vi "Logger.Stats.UpdateGraph.vi"(8 "error in (no error)":errorcluster, 9 "Selection":i32[](array[numeric]), 10 "Results":T1[](array[typedef]) {"Time From" format="%<%X %x>T"; "Time To" format="%<%X %x>T"}, 11 "Graph":refnum<vi>) -> (0 "error out":errorcluster)   [LabVIEW 2016]
uses:
  Logger.Stats.Fglb.Result.ctl
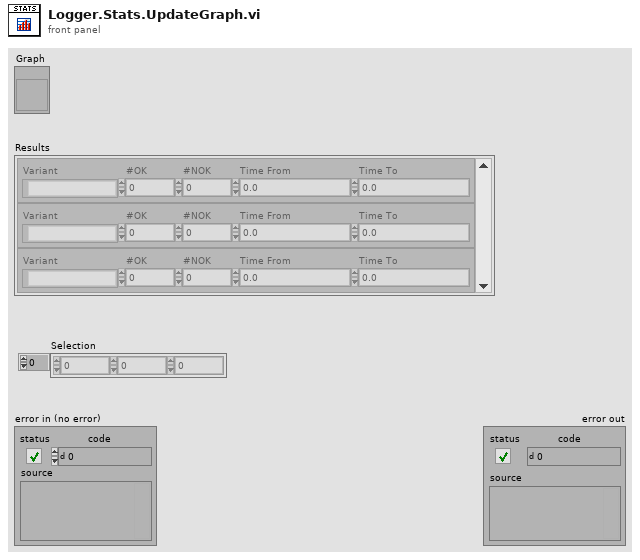
[diagram p1: front panel]
types:
  T1 = typedef "Logger.Stats.Fglb.Result.ctl" = cluster{"Variant":string, "#OK":i32, "#NOK":i32, "Time From":dbl, "Time To":dbl}
  T2 = cluster{"Name":string, "Color":u32, "Style":i32, "Point Style":i32, "Name Visible":bool, "Allow Drag":bool, "Annotation Mode":u32, "Plot":i32, "Index":i32, "Position":cluster{"X":dbl, "Y":dbl}, "X Scale":i32, "Y Scale":u32, "Show Arrow":bool, "Lock Name":bool, "Plot Area":i32, "Label Offset":cluster{"X":dbl, "Y":i32}}
  T3 = cluster{"Name":string, "Color":u32, "Style":i32, "Point Style":i32, "Name Visible":bool, "Allow Drag":bool, "Annotation Mode":u32, "Plot":i32, "Index":i32, "Position":cluster{"X":dbl, "Y":dbl}, "X Scale":i32, "Y Scale":u32, "Show Arrow":bool, "Lock Name":bool, "Plot Area":i32, "Label Offset":cluster{"X":dbl, "Y":i32}}[]
  T4 = typedef "LVAnnotationListTypeDef.ctl" = cluster{"Name":string, "Color":u32, "Style":u8, "Point Style":u8, "Name Visible":bool, "Allow Drag":bool, "Annotation Mode":u32, "Plot":i32, "Index":i32, "Position":cluster{"X":dbl, "Y":dbl}, "X Scale":u32, "Y Scale":u32, "Show Arrow":bool, "Lock Name":bool, "Plot Area":i32, "Label Offset":cluster{"X":dbl, "Y":dbl}}[]
  T5 = cluster{"Name":string, "Color":u32, "Style":u8, "Point Style":u8, "Name Visible":bool, "Allow Drag":bool, "Annotation Mode":u32, "Plot":i32, "Index":i32, "Position":cluster{"X":dbl, "Y":dbl}, "X Scale":u32, "Y Scale":u32, "Show Arrow":bool, "Lock Name":bool, "Plot Area":i32, "Label Offset":cluster{"X":dbl, "Y":dbl}}
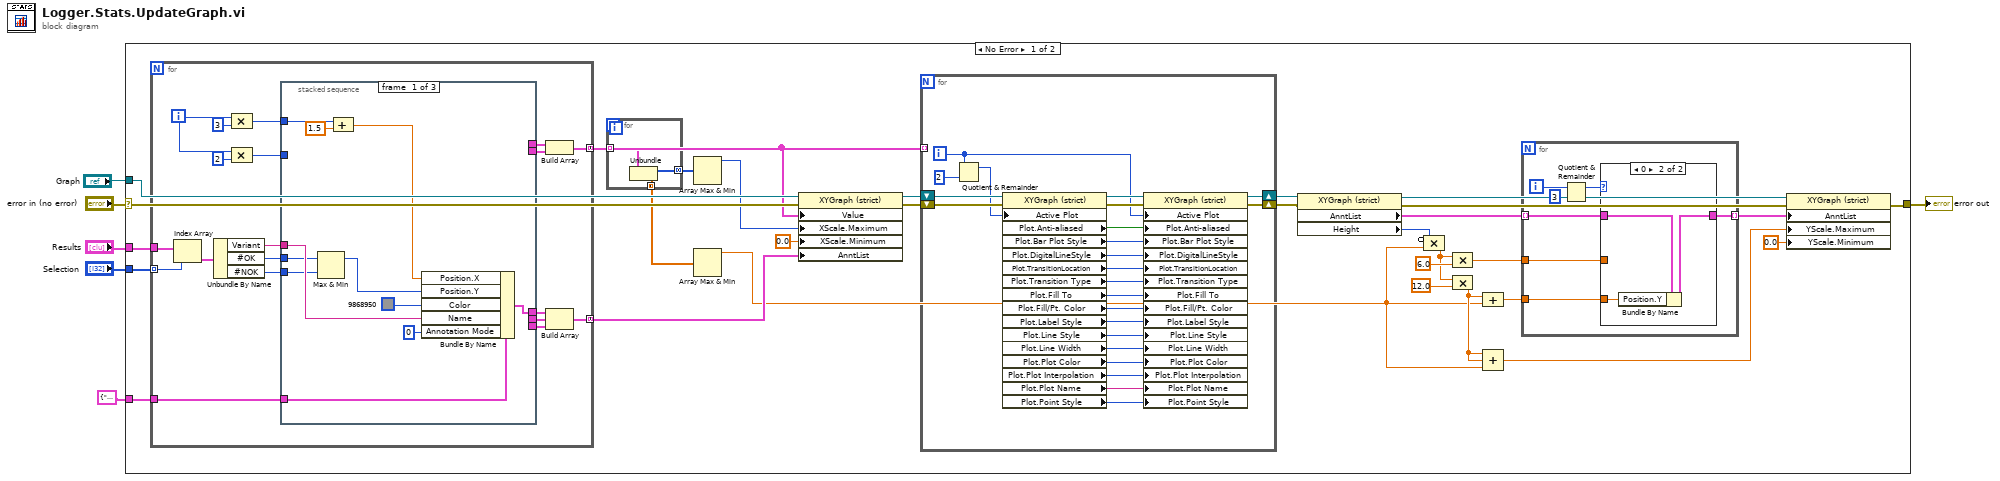
[diagram p0: block diagram]
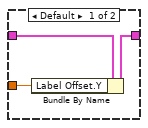
[diagram p2: hidden frame]
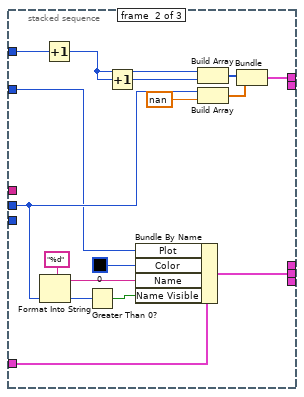
[diagram p3: hidden frame]
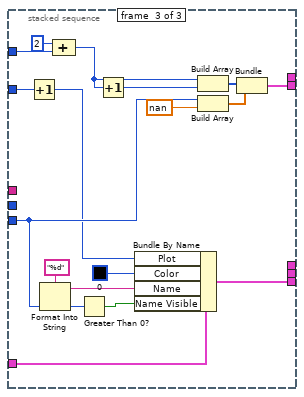
[diagram p4: hidden frame]
diagram:
  n1 = case shown="No Error" "error in (no error)" {
    selector: "error in (no error)" -> [w34 w138]
    tunnel: [w24 w138] -> w5
    tunnel: "Results" -> [w36 _]
    tunnel: "Graph" -> [w33 _]
    tunnel: "Selection" -> [w35 _]
    tunnel: T2 {"Name"="", "Color"=0, "Style"=0, "Point Style"=0, "Name Visible"=TRUE, "Allow Drag"=FALSE, "Annotation Mode"=1, "Plot"=0, "Index"=0, "Position"={"X"=0.0, "Y"=0.0}, "X Scale"=0, "Y Scale"=0, "Show Arrow"=FALSE, "Lock Name"=TRUE, "Plot Area"=0, "Label Offset"={"X"=0.0, "Y"=0}} ("Cluster") -> [w32 _]
    frame No Error {
      n2 = for {
        tunnel: w36 -> [w68]
        tunnel: w35 -> [w67] mode=indexing
        tunnel: w32 -> [w63]
        tunnel: [w55] -> w30 mode=concatenating
        tunnel: [w56] -> w25 mode=concatenating
        i -> [w52]
        n3 = Index Array(array=w68, index=w67) -> (element=w66:T1)
        n4 = Unbundle By Name(w66) -> ("Variant"=w57:string, "#OK"=w64:i32, "#NOK"=w54:i32)
        n5 = Compound Arithmetic op=MULTIPLY(w52, 3 ("value")) -> (w62:i32)
        n6 = Compound Arithmetic op=MULTIPLY(w52, 2 ("value")) -> (w51:i32)
        n7 = stacked-sequence {
          tunnel: w64 -> [w71 w83 _]
          tunnel: w54 -> [w70 _ w101]
          tunnel: w63 -> [w78 w93 w110]
          tunnel: w62 -> [w74 w90 w97]
          tunnel: [_ w85 _] -> w60
          tunnel: [_ w84 _] -> w61
          tunnel: [_ _ w104] -> w59
          tunnel: [_ _ w103] -> w58
          tunnel: w57 -> [w77 _ _]
          tunnel: w51 -> [_ w80 w99]
          tunnel: [w76 _ _] -> w50
          frame #0 {
            n8 = Max & Min(x=w71, y=w70) -> (max(x,y)=w69:i32)  [unwired: 1 out]
            n9 = Compound Arithmetic op=unknown(w74, 1.5 ("value")) -> (w72:dbl)
            n10 = Bundle By Name(cluster=w78, "Position.X"=w72, "Position.Y"=w69, "Color"=u32 9868950, "Name"=w77, "Annotation Mode"=u32 0) -> (w76:T2)
          }
          frame #1 {
            n11 = Format Into String(format string="%d", w83) -> (resulting string=w91:string)  [unwired: 2 in, 1 out]
            n12 = Increment(x=w90) -> (x+1=w81:i32)
            n13 = Greater Than 0?(x=w83) -> (x > 0?=w82:bool)
            n14 = Increment(x=w81) -> (x+1=w89:i32)
            n15 = Bundle By Name(cluster=w93, "Plot"=w80, "Color"=u32 0, "Name"=w91, "Name Visible"=w82) -> (w84:T2)
            n16 = Build Array(w81, w89) -> (w87:i32[])
            n17 = Build Array(w83, nan ("element")) -> (w86:dbl[])
            n18 = Bundle(w87, w86) -> (w85:cluster{i32[], dbl[]})  [unwired: 1 in]
          }
          frame #2 {
            n19 = Increment(x=w99) -> (x+1=w98:i32)
            n20 = Format Into String(format string="%d", w101) -> (resulting string=w108:string)  [unwired: 2 in, 1 out]
            n21 = Compound Arithmetic op=ADD(2 ("value"), w97) -> (w95:i32)
            n22 = Greater Than 0?(x=w101) -> (x > 0?=w102:bool)
            n23 = Increment(x=w95) -> (x+1=w100:i32)
            n24 = Bundle By Name(cluster=w110, "Plot"=w98, "Color"=u32 0, "Name"=w108, "Name Visible"=w102) -> (w103:T2)
            n25 = Build Array(w95, w100) -> (w106:i32[])
            n26 = Build Array(w101, nan ("element")) -> (w105:dbl[])
            n27 = Bundle(w106, w105) -> (w104:cluster{i32[], dbl[]})  [unwired: 1 in]
          }
        }
        n28 = Build Array(w60, w59) -> (w55:cluster{i32[], dbl[]}[])
        n29 = Build Array(w50, w61, w58) -> (w56:T3)
      }
      n30 = for {
        tunnel: w30 -> [w114] mode=indexing
        tunnel: [w113] -> w31 mode=concatenating
        tunnel: [w112] -> w8 mode=concatenating
        n31 = Unbundle(w114) -> (w113:i32[], w112:dbl[])
      }
      n32 = Array Max & Min(array=w31) -> (max value=w10:i32)  [unwired: 3 out]
      n33 = Array Max & Min(array=w8) -> (max value=w7:dbl)  [unwired: 3 out]
      n34 = property class="XYGraph (strict)"(reference=w33, error in=w34, "Value"=w30, "XScale.Maximum"=w10, "XScale.Minimum"=0.0 ("X Scale.Range:Minimum"), "AnntList"=w25) -> (reference out=w28:refnum<vi>, error out=w29:errorcluster)
      n35 = for {
        tunnel: w30 -> [_] mode=indexing
        shift-right: [w116] -> w27
        shift-left: w29 -> [w136]
        shift-right: [w115] -> w26
        shift-left: w28 -> [w137]
        i -> [w119]
        n36 = Quotient & Remainder(x=w119, y=2) -> (x-y*floor(x/y)=w117:i32)  [unwired: 1 out]
        n37 = property class="XYGraph (strict)"(reference=w137, error in=w136, "Active Plot"=w117) -> (reference out=w135:refnum<vi>, error out=w134:errorcluster, "Plot.Anti-aliased"=w133:bool, "Plot.Bar Plot Style"=w132:u8, "Plot.DigitalLineStyle"=w131:u8, "Plot.TransitionLocation"=w130:u8, "Plot.Transition Type"=w129:u8, "Plot.Fill To"=w128:i16, "Plot.Fill/Pt. Color"=w127:u32, "Plot.Label Style"=w126:u8, "Plot.Line Style"=w125:u8, "Plot.Line Width"=w124:u8, "Plot.Plot Color"=w123:u32, "Plot.Plot Interpolation"=w120:u8, "Plot.Plot Name"=w121:string, "Plot.Point Style"=w122:u8)
        n38 = property class="XYGraph (strict)"(reference=w135, error in=w134, "Active Plot"=w119, "Plot.Anti-aliased"=w133, "Plot.Bar Plot Style"=w132, "Plot.DigitalLineStyle"=w131, "Plot.TransitionLocation"=w130, "Plot.Transition Type"=w129, "Plot.Fill To"=w128, "Plot.Fill/Pt. Color"=w127, "Plot.Label Style"=w126, "Plot.Line Style"=w125, "Plot.Line Width"=w124, "Plot.Plot Color"=w123, "Plot.Plot Interpolation"=w120, "Plot.Plot Name"=w121, "Plot.Point Style"=w122) -> (reference out=w115:refnum<vi>, error out=w116:errorcluster)
      }
      n39 = property class="XYGraph (strict)"(reference=w26, error in=w27) -> (reference out=w21:refnum<vi>, error out=w22:errorcluster, "AnntList"=w23:T4, "Height"=w19:u32)
      n40 = Compound Arithmetic op=MULTIPLY(invert w19, w7) -> (w15:dbl)
      n41 = Compound Arithmetic op=MULTIPLY(w15, 6.0 ("value")) -> (w16:dbl)
      n42 = Compound Arithmetic op=MULTIPLY(w15, 12.0 ("value")) -> (w14:dbl)
      n43 = Compound Arithmetic op=ADD(w14, w7) -> (w13:dbl)
      n44 = Compound Arithmetic op=ADD(w14, w14, w7) -> (w12:dbl)
      n45 = for {
        tunnel: w23 -> [w43] mode=indexing
        tunnel: [w42] -> w20 mode=indexing
        tunnel: w16 -> [w38]
        tunnel: w13 -> [w37]
        i -> [w40]
        n46 = Quotient & Remainder(x=w40, y=3) -> (x-y*floor(x/y)=w39:i32)  [unwired: 1 out]
        n47 = case shown="0" w39 {
          tunnel: w43 -> [w46 w49]
          tunnel: [w45 w48] -> w42
          tunnel: w38 -> [w44 _]
          tunnel: w37 -> [_ w47]
          frame Default {
            n48 = Bundle By Name(cluster=w46, "Label Offset.Y"=w44) -> (w45:T5)
          }
          frame 0 {
            n49 = Bundle By Name(cluster=w49, "Position.Y"=w47) -> (w48:T5)
          }
        }
      }
      n50 = property class="XYGraph (strict)"(reference=w21, error in=w22, "AnntList"=w20, "YScale.Maximum"=w12, "YScale.Minimum"=0.0 ("Y Scale.Range:Minimum")) -> (error out=w24:errorcluster)  [unwired: 1 out]
    }
    frame Error {
    }
  }
  "error out" <- w5
